vi "emi_Default Ini File Name.vi"(7 "Name":string, 11 "error in (no error)":errorcluster) -> (8 "Path":path, 15 "error out":errorcluster)   [LabVIEW 2011]
doc: "On error, no change\n\nRetreive default ini file path. uses /config/config.ini as default"
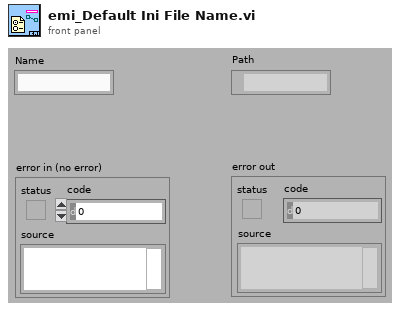
[diagram p1: front panel]
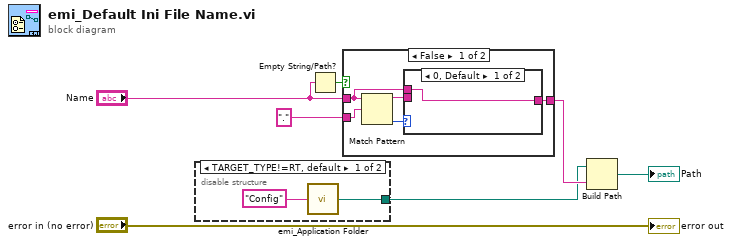
[diagram p0: block diagram]
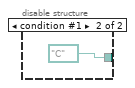
[diagram p2: hidden frame]
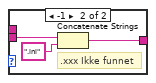
[diagram p3: hidden frame]
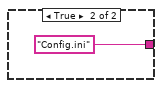
[diagram p4: hidden frame]
diagram:
  n1 = disable-structure shown="TARGET_TYPE!=RT, default" {
    disable-tunnel: [w8 path "C:/" ("Dir")] -> w1
    frame condition #0 (active) {
      n2 = call "emi_Application Folder.vi"("Sub Dir name"="Config") -> ("Dir"=w8:path)  [unwired: 13 in, 1 out]
    }
    frame condition #1 {
    }
  }
  n3 = Empty String/Path?(string/path="Name") -> (empty?=w3:bool)
  n4 = case shown="False" w3 {
    tunnel: "." -> [w15 _]
    tunnel: "Name" -> [w13 _]
    tunnel: [w11 "Config.ini" ("Name")] -> w6
    frame False {
      n5 = Match Pattern(string=w13, regular expression=w15) -> (before substring=w12:string, offset past match=w14:i32)  [unwired: 1 in, 2 out]
      n6 = case shown="0, Default" w14 {
        tunnel: w13 -> [w16 _]
        tunnel: w12 -> [_ w19]
        tunnel: [w16 w17] -> w11
        frame 0, Default {
        }
        frame -1 {
          # ".xxx Ikke funnet"
          n7 = Concatenate Strings(w19, ".ini") -> (w17:string)
        }
      }
    }
    frame True {
    }
  }
  n8 = Build Path(base path=w1, name or relative path=w6) -> (appended path=→"Path":path)
  "error out" <- "error in (no error)"
